vi "UpdateCVT.vi"(8 "error in":errorcluster, 11 "MetaDriver_v1 in":refnum<class "MetaDriver_v1.lvclass">) -> (0 "error out":errorcluster, 3 "MetaDriver_v1 out":refnum<class "MetaDriver_v1.lvclass">)   [LabVIEW 2013, in "MetaDriver_v1.lvclass"]
doc: "This method sets the CVT value of a single Property.\n\nCompatible with the following properties:\n\nEnum\nNumeric\nString/Path\nCluster of Numerics where the current value is a numeric labelled 'Value' (Choiche1.ctl)\n\nIT DOES NOT WORK WITH NESTED CLUSTERS OR ARRAYS"
uses:
  MetaDriver_v1.lvclass
panel:
  out "error in":errorcluster
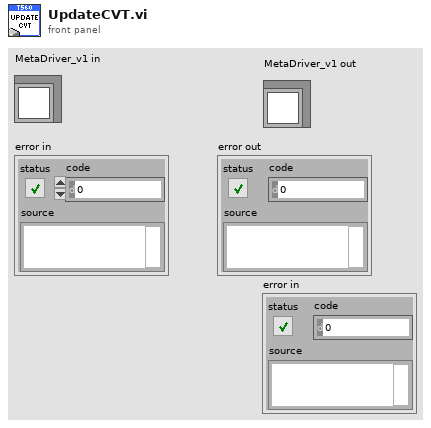
[diagram p1: front panel]
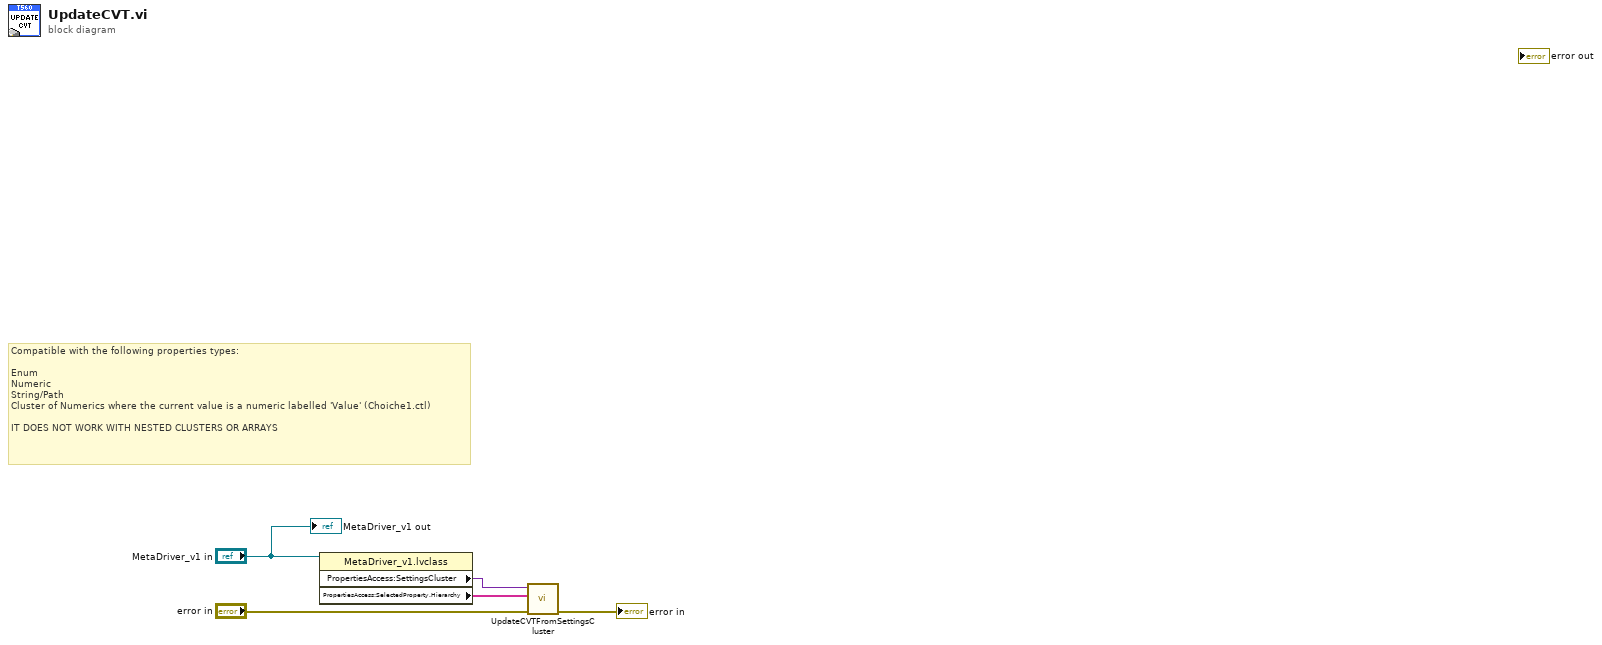
[diagram p0: block diagram]
diagram:
  # "Compatible with the following properties types:\n\nEnum\nNumeric\nString/Path\nCluster of Numerics where the current value is a numeric labelled 'Value' (Choiche1.ctl)\n\nIT DOES NOT WORK WITH NESTED CLUSTERS OR ARRAYS"
  n1 = property class="MetaDriver_v1.lvclass"(reference="MetaDriver_v1 in") -> ("PropertiesAccess:SettingsCluster"=w1:variant, "PropertiesAccess:SelectedProperty.Hierarchy"=w2:string[])  [unwired: 1 in, 2 out]
  n2 = call "UpdateCVTFromSettingsCluster.vi"("error in"="error in", "SelectedProperty.Hierarchy"=w2, "SettingsCluster"=w1) -> ("error out"=→"error in":errorcluster)  [unwired: 8 in]
  "MetaDriver_v1 out" <- "MetaDriver_v1 in"
